vi "Read WPC Player Stat File.vi"(11 "file path (use dialog)":path=path "C:/Users/manma/Google Drive/WPC Stat Scrape/Data/WPC Stats.bin") -> (0 "error out":errorcluster, 2 "Latest WPC Stats":T1[](array[typedef]) {"Date Updated" format="%<%m/%d/%Y>T"}, 3 "Full WPC Stats":T1[][](array[typedef]) {"Date Updated" format="%<%m/%d/%Y>T"})   [LabVIEW 2021]
uses:
  WPC Player and Financial Stats.ctl
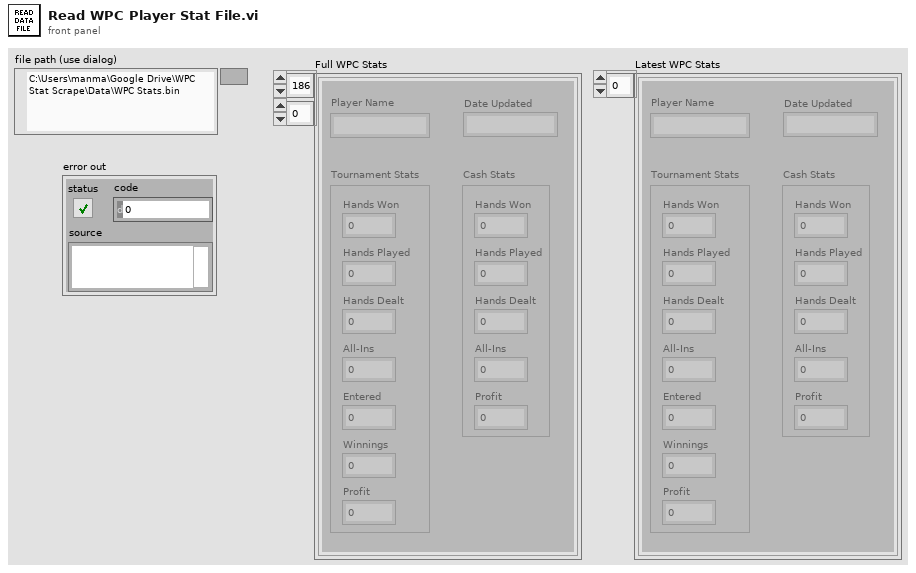
[diagram p1: front panel]
types:
  T1 = typedef "WPC Player and Financial Stats.ctl" = cluster{"Player Name":string, "Date Updated":timestamp, "Tournament Stats":cluster{"Hands Won":i32, "Hands Played":i32, "Hands Dealt":i32, "All-Ins":i32, "Entered":i32, "Winnings":dbl, "Profit":dbl}, "Cash Stats":cluster{"Hands Won":i32, "Hands Played":i32, "Hands Dealt":i32, "All-Ins":i32, "Profit":dbl}}
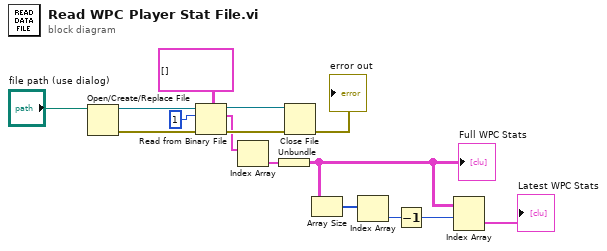
[diagram p0: block diagram]
diagram:
  n1 = Open/Create/Replace File(file path (use dialog)="file path (use dialog)") -> (refnum out=w14:refnum<file>, error out=w13:errorcluster)  [unwired: 5 in, 1 out]
  n2 = Read from Binary File(5:T1[][] [], 8:w13, 10:1 ("count (1)"), 11:w14) -> (0:w11:errorcluster, 2:w8:cluster{T1[][]}[], 3:w10:refnum<file>)  [unwired: 2 in, 1 out]
  n3 = Index Array(array=w8) -> (element=w7:cluster{T1[][]})  [unwired: 1 in]
  n4 = Unbundle(w7) -> (w4:T1[][])
  "Full WPC Stats" <- w4
  n5 = Close File(refnum=w10, error in=w11) -> (error out=→"error out":errorcluster)  [unwired: 1 out]
  n6 = Array Size(array=w4) -> (size(s)=w5:i32[])
  n7 = Index Array(array=w5) -> (element=w3:i32)  [unwired: 1 in]
  n8 = Decrement(x=w3) -> (x-1=w2:i32)
  n9 = Index Array(array=w4, index (row)=w2) -> (element=→"Latest WPC Stats":T1[])  [unwired: 1 in]
